vi "Utility Multiple Write To Registers.vi"(0 "VISA resource name":refnum<visa-resource-name>, 1 "Unit Address (1)":u8=1, 5 "Registers Addresses (0)":u16[](array[numeric])=[21, 123, 124, 54, 128], 7 "Data (0)":i16[](array[numeric]), 11 "error in (no error)":errorcluster) -> (4 "VISA resource name out":refnum<visa-resource-name>, 15 "error out":errorcluster)   [LabVIEW 2014, in "Eurotherm 35xx Series.lvlib"]
doc: "This VI writes the values to the specified registers of specified unit."
uses:
  <instrlib>/Eurotherm 35xx Series/Eurotherm 35xx Series.lvlib
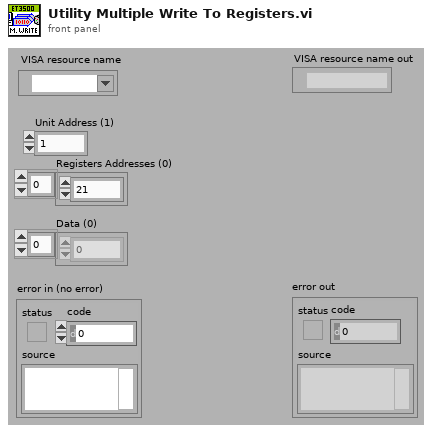
[diagram p1: front panel]
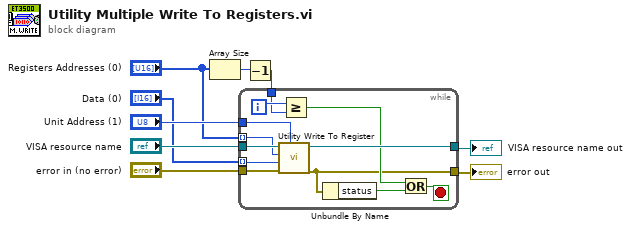
[diagram p0: block diagram]
diagram:
  n1 = Array Size(array="Registers Addresses (0)") -> (size(s)=w7:i32)
  n2 = Decrement(x=w7) -> (x-1=w6:i32)
  n3 = while {
    tunnel: [w21] -> w9
    tunnel: [w16] -> w8
    tunnel: w6 -> [w15]
    tunnel: "Unit Address (1)" -> [w14]
    tunnel: "error in (no error)" -> [w13]
    tunnel: "VISA resource name" -> [w12]
    tunnel: "Registers Addresses (0)" -> [w11] mode=indexing
    tunnel: "Data (0)" -> [w10] mode=indexing
    i -> [w20]
    stop <- w19 stop-if-true
    n4 = call <instrlib>:"Utility Write To Register.vi"("Unit Address (1)"=w14, "error in (no error)"=w13, "Data (0)"=w10, "Register Address (0)"=w11, "VISA resource name"=w12) -> ("error out"=w16:errorcluster, "VISA resource name out"=w21:refnum<visa-resource-name>)  [unwired: 5 in]
    n5 = Greater Or Equal?(x=w20, y=w15) -> (x >= y?=w17:bool)
    n6 = Unbundle By Name(w16) -> ("status"=w18:bool)
    n7 = Or(x=w17, y=w18) -> (x .or. y?=w19:bool)
  }
  "error out" <- w8
  "VISA resource name out" <- w9
